vi "Tell Parent.vi"(4 "Priority":bool, 7 "Actor in":refnum<class "Actor.lvclass">, 10 "Msg":refnum<class "Msg.lvclass">) -> (0 "Error out":errorcluster)   [LabVIEW 2025, in "jettl.lvlib"]
uses:
  jettl.lvlib
  Relation.ctl
  Teller/Teller.lvlib
  Actor/Actor.lvclass
  Attributes/Attributes/Attributes.lvclass
  Transport/Transport/Transport.lvclass
  Msg/Msg.lvclass
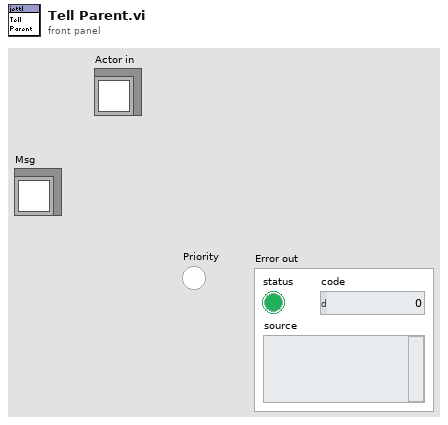
[diagram p1: front panel]
types:
  T1 = typedef "jettl.lvlib/Relation.ctl" = enum16{"Self", "Parent", "Child"}
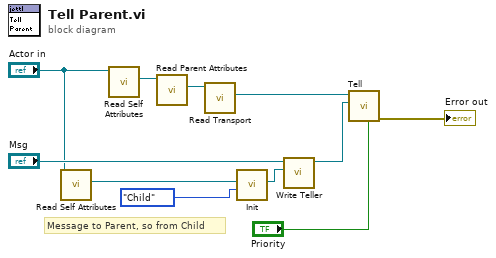
[diagram p0: block diagram]
diagram:
  # "Message to Parent, so from Child"
  n1 = call-dynamic "Read Self Attributes.vi"("Actor in"="Actor in") -> ("Self Attributes"=w8:refnum<class "Attributes.lvclass">)  [unwired: 10 in]
  n2 = call-dynamic "Read Self Attributes.vi"("Actor in"="Actor in") -> ("Self Attributes"=w3:refnum<class "Attributes.lvclass">)  [unwired: 10 in]
  n3 = call-dynamic "Read Parent Attributes.vi"("Attributes in"=w3) -> ("Parent Attributes"=w2:refnum<class "Attributes.lvclass">)  [unwired: 10 in]
  n4 = call-dynamic "Read Transport.vi"("Attributes in"=w2) -> ("Transport"=w6:refnum<class "Transport.lvclass">)  [unwired: 10 in]
  n5 = call "Init.vi"("Relation"=Relation."Child", "Self Attributes"=w8) -> ("Teller"=w9:refnum<class "Teller.lvclass">)  [unwired: 9 in]
  n6 = call-dynamic "Write Teller.vi"("Teller"=w9, "Msg in"="Msg") -> ("Msg out"=w5:refnum<class "Msg.lvclass">)  [unwired: 9 in]
  n7 = call-dynamic "Tell.vi"("Priority"="Priority", "Msg"=w5, "Transport in"=w6) -> ("Error out"=→"Error out":errorcluster)  [unwired: 8 in]
